vi "InAs-GaAs superlattice-111229a.vi"() -> ()   [LabVIEW 2011]
uses:
  development/wait_globals.vi
panel:
  out "Wait Time Remaining(m:s)":string
  out "Waiting":bool
  out "Total Wait Time (m:s)":string
  out "step number  5":i32
  in  "Number of \nGrowth Steps 5":i32=10
  out "step number  4":i32
  in  "Number of \nGrowth Steps 4":i32=10
  out "step number  3":i32
  in  "Number of \nGrowth Steps 3":i32=10
  out "step number  2":i32
  in  "Number of \nGrowth Steps 2":i32=10
  in  "Ga Flow 1":dbl=5.49
  in  "Indium Flow":dbl=45.0
  in  "Number of \nGrowth Steps":i32=10
  out "step number":i32
  in  "As_Gas Flow":dbl=3.4
  in  "Manifold H2 Flow":dbl=730.0
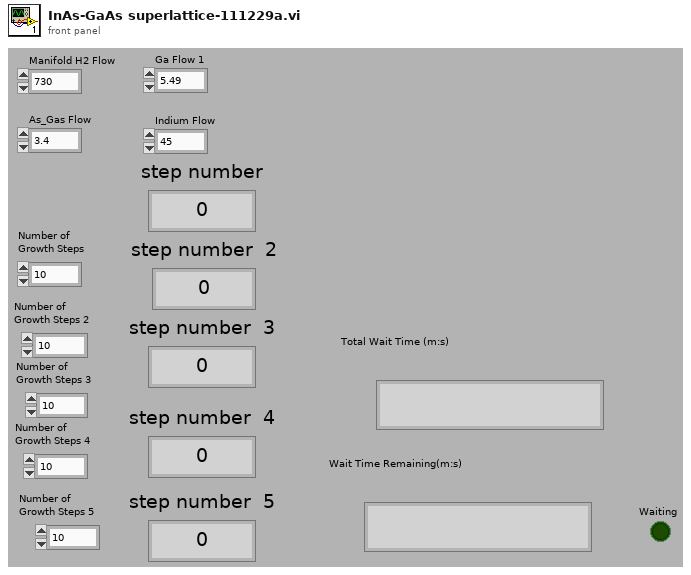
[diagram p1: front panel]
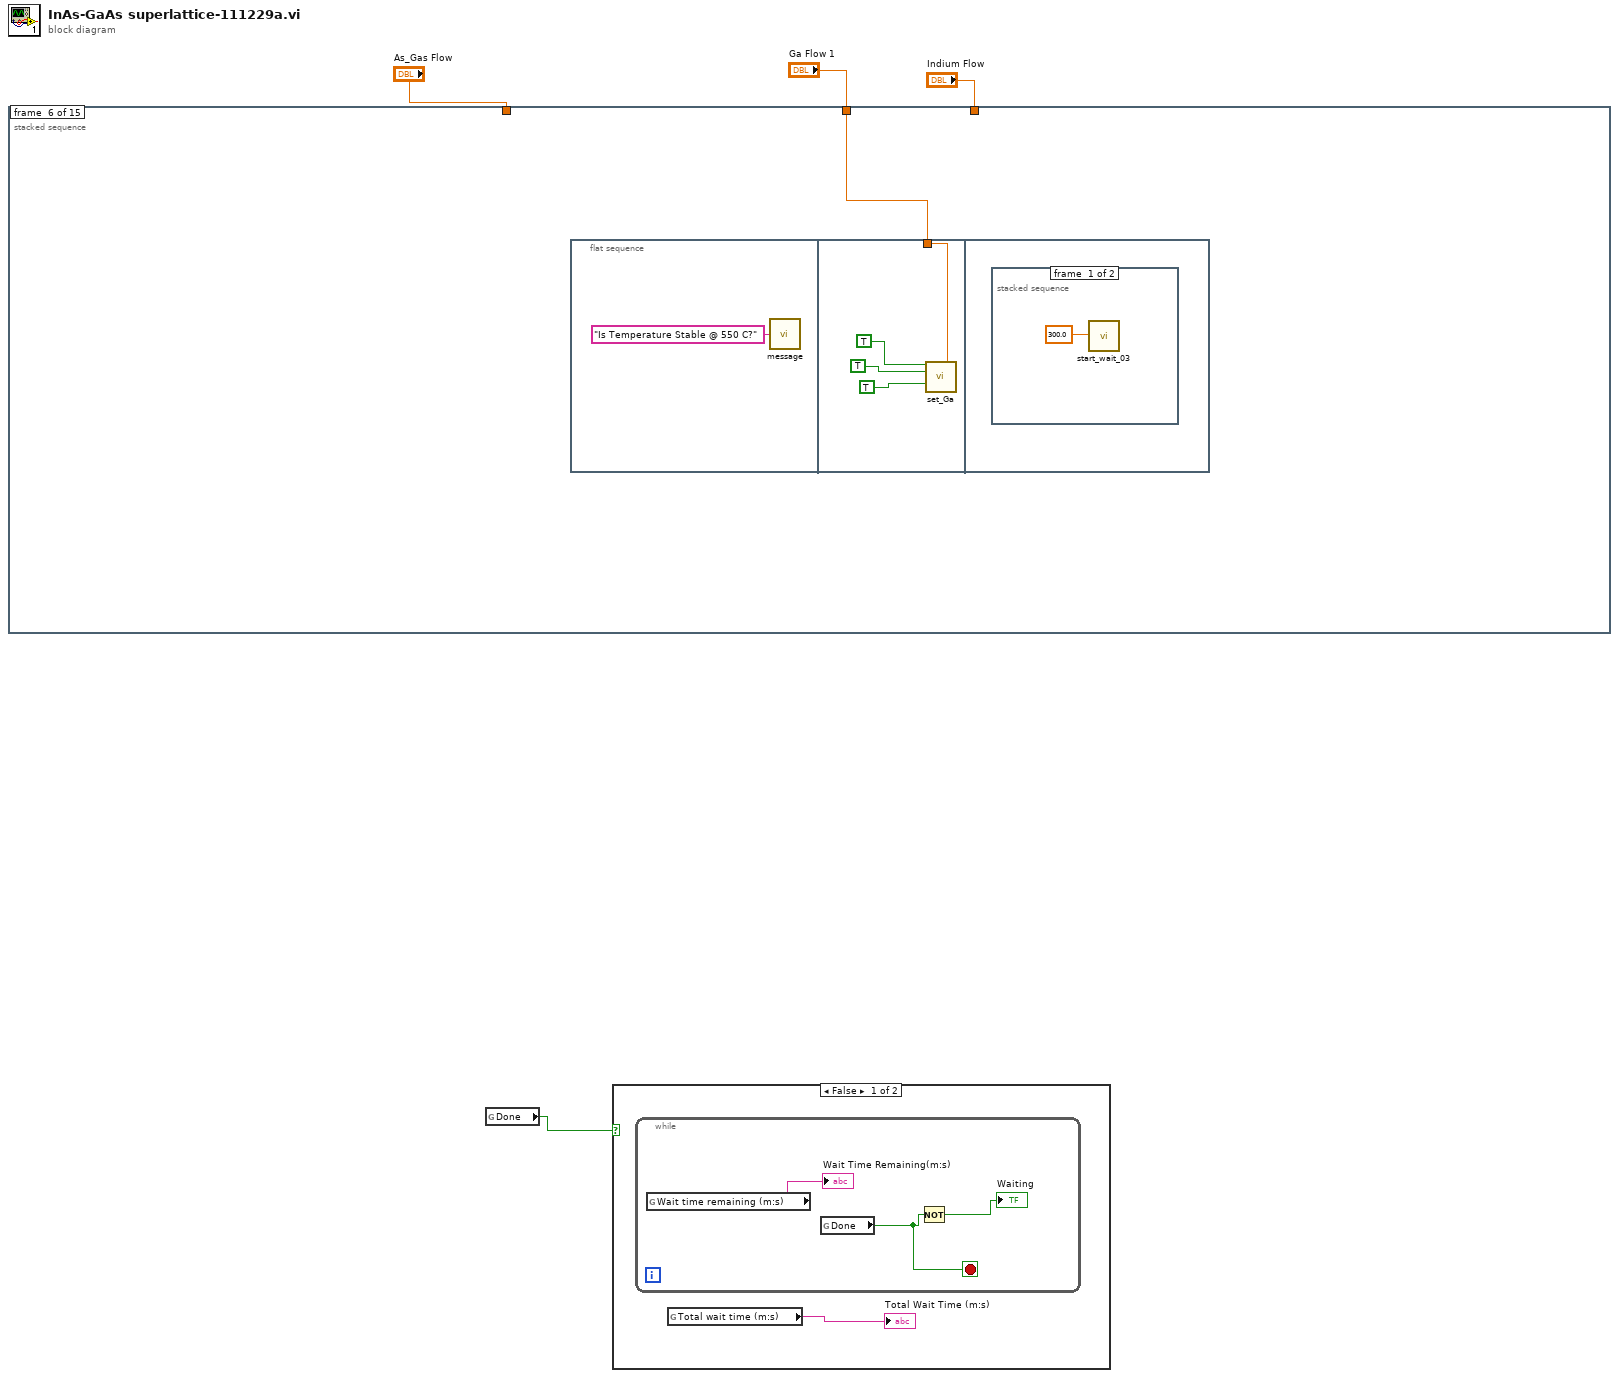
[diagram p0: block diagram]
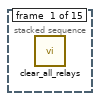
[diagram p3: hidden frame]
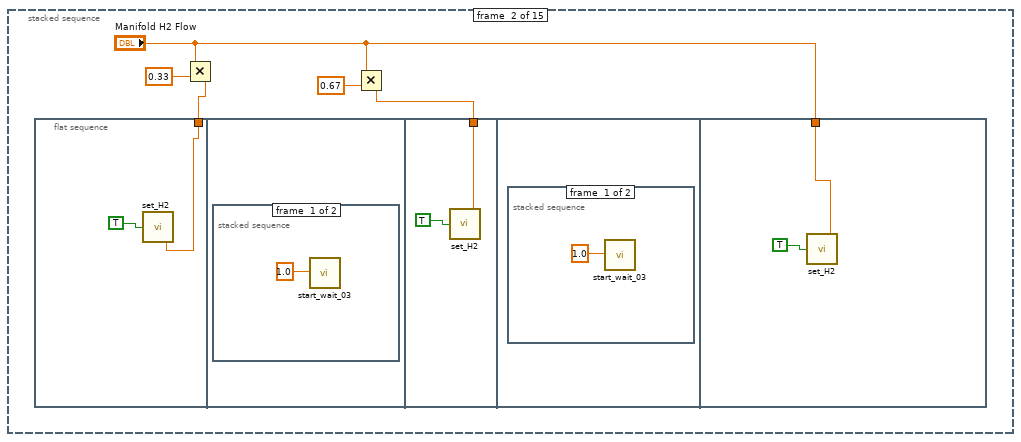
[diagram p4: hidden frame]
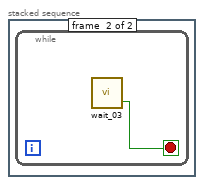
[diagram p5: hidden frame]
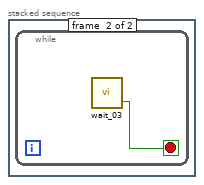
[diagram p6: hidden frame]
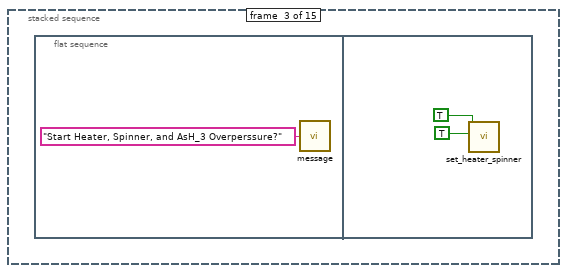
[diagram p7: hidden frame]
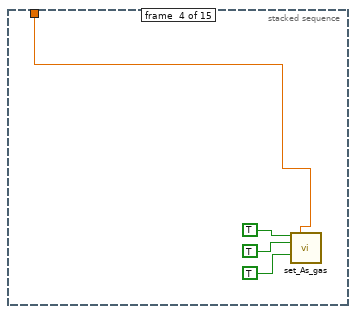
[diagram p8: hidden frame]
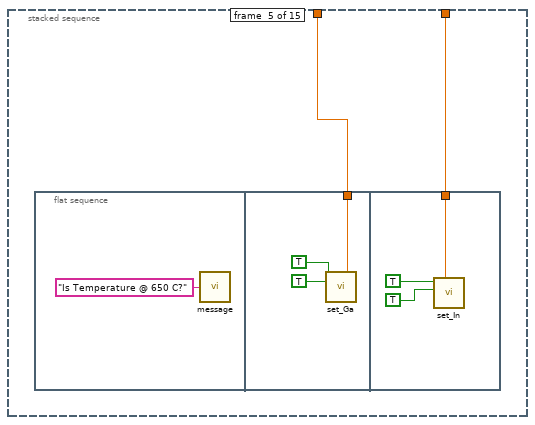
[diagram p9: hidden frame]
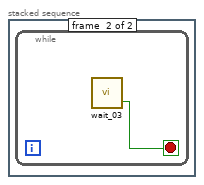
[diagram p10: hidden frame]
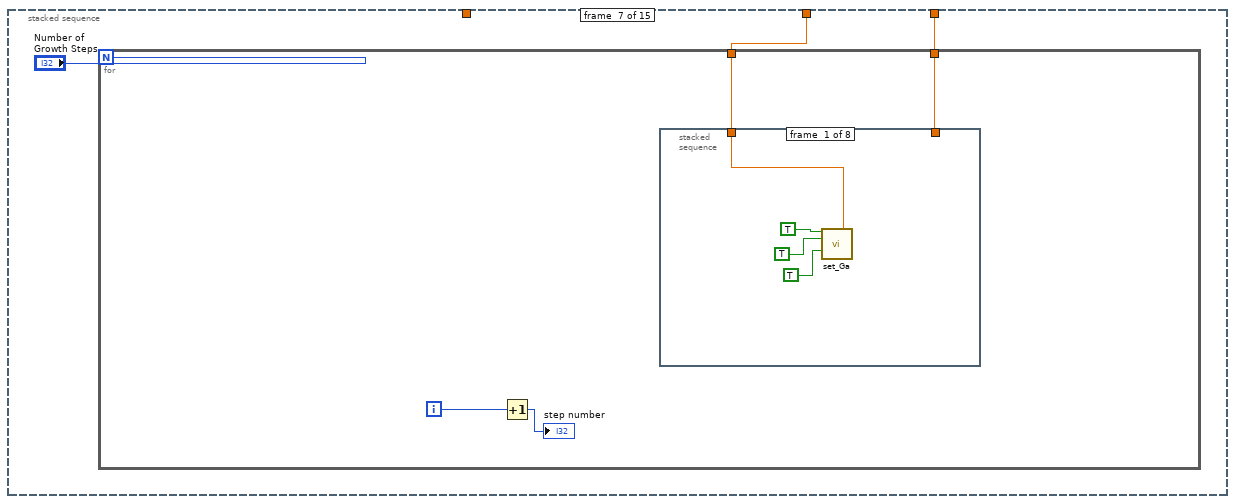
[diagram p11: hidden frame]
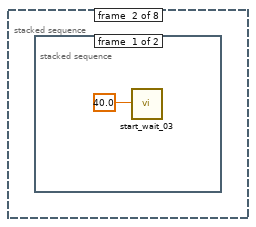
[diagram p12: hidden frame]
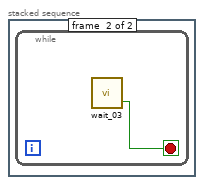
[diagram p13: hidden frame]
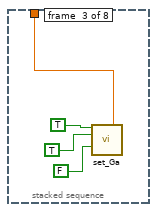
[diagram p14: hidden frame]
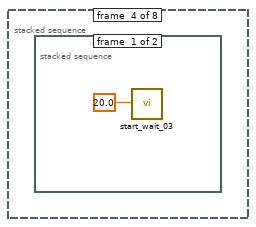
[diagram p15: hidden frame]
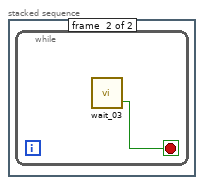
[diagram p16: hidden frame]
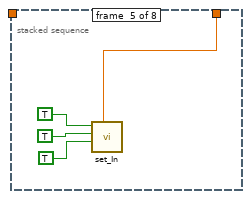
[diagram p17: hidden frame]
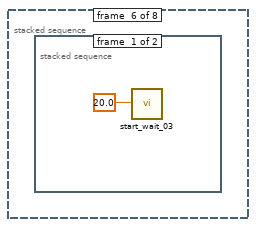
[diagram p18: hidden frame]
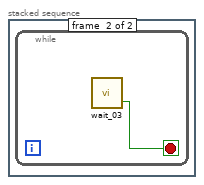
[diagram p19: hidden frame]
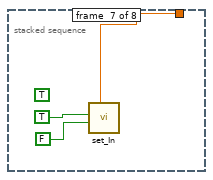
[diagram p20: hidden frame]
diagram:
  n1 = stacked-sequence {
    tunnel: "Ga Flow 1" -> [_ _ _ _ w28 w36 w45 w75 w105 w135 w165 _ _ _ _]
    tunnel: "As_Gas Flow" -> [_ _ _ w23 _ _ _ _ _ _ _ _ _ _ _]
    tunnel: "Indium Flow" -> [_ _ _ _ w27 _ w44 w74 w104 w134 w164 _ _ _ _]
    frame #0 {
      n2 = call "clear_all_relays.vi"() -> ()  [unwired: 2 out]
    }
    frame #1 {
      n3 = flat-sequence {
        tunnel: w9 -> [w10]
        tunnel: w7 -> [w14]
        tunnel: "Manifold H2 Flow" -> [w18]
        frame #0 {
          n4 = call "set_H2.vi"("Manifold H2 Flow"=w10, "H2 Active"=TRUE) -> ()  [unwired: 2 in, 2 out]
        }
        frame #1 {
          n5 = stacked-sequence {
            frame #0 {
              n6 = call "start_wait_03.vi"("Total wait time (s)"=1.0 ("Wait (s)")) -> ()
            }
            frame #1 {
              n7 = while {
                stop <- w13 stop-if-true
                n8 = call "wait_03.vi"() -> ("Done"=w13:bool)  [unwired: 1 in, 1 out]
              }
            }
          }
        }
        frame #2 {
          n9 = call "set_H2.vi"("Manifold H2 Flow"=w14, "H2 Active"=TRUE) -> ()  [unwired: 2 in, 2 out]
        }
        frame #3 {
          n10 = stacked-sequence {
            frame #0 {
              n11 = call "start_wait_03.vi"("Total wait time (s)"=1.0 ("Wait (s)")) -> ()
            }
            frame #1 {
              n12 = while {
                stop <- w17 stop-if-true
                n13 = call "wait_03.vi"() -> ("Done"=w17:bool)  [unwired: 1 in, 1 out]
              }
            }
          }
        }
        frame #4 {
          n14 = call "set_H2.vi"("Manifold H2 Flow"=w18, "H2 Active"=TRUE) -> ()  [unwired: 2 in, 2 out]
        }
      }
      n15 = Multiply(x="Manifold H2 Flow", y=0.33) -> (x*y=w9:dbl)
      n16 = Multiply(x="Manifold H2 Flow", y=0.67) -> (x*y=w7:dbl)
    }
    frame #2 {
      n17 = flat-sequence {
        frame #0 {
          n18 = call "message.vi"("message"="Start Heater, Spinner, and AsH_3 Overperssure?") -> ()
        }
        frame #1 {
          n19 = call "set_heater_spinner.vi"("Spinner"=TRUE, "Heater"=TRUE) -> ()  [unwired: 1 in, 7 out]
        }
      }
    }
    frame #3 {
      n20 = call "set_As_gas.vi"("As_Gas Active"=TRUE, "As_Gas Flow"=w23, "As_Gas In"=TRUE, "As_Gas Run"=TRUE) -> ()  [unwired: 2 in, 10 out]
    }
    frame #4 {
      n21 = flat-sequence {
        tunnel: w28 -> [w30]
        tunnel: w27 -> [w33]
        frame #0 {
          n22 = call "message.vi"("message"="Is Temperature @ 650 C?") -> ()
        }
        frame #1 {
          n23 = call "set_Ga.vi"("Ga Active"=TRUE, "Ga Flow 1"=w30, "Ga Bubbler"=TRUE) -> ()  [unwired: 5 in, 8 out]
        }
        frame #2 {
          n24 = call "set_In.vi"("Indium Flow"=w33, "In Bubbler"=TRUE ("Ga Bubbler"), "In Active"=TRUE ("Ga Active")) -> ()  [unwired: 2 in, 5 out]
        }
      }
    }
    frame #5 {
      n25 = flat-sequence {
        tunnel: w36 -> [w38]
        frame #0 {
          n26 = call "message.vi"("message"="Is Temperature Stable @ 550 C?") -> ()
        }
        frame #1 {
          n27 = call "set_Ga.vi"("Ga Active"=TRUE ("P_Gas Active"), "Ga Flow 1"=w38, "Ga Bubbler"=TRUE ("P_Gas In"), "Ga Run"=TRUE ("P_Gas Run")) -> ()  [unwired: 4 in, 8 out]
        }
        frame #2 {
          n28 = stacked-sequence {
            frame #0 {
              n29 = call "start_wait_03.vi"("Total wait time (s)"=300.0 ("Wait (s)")) -> ()
            }
            frame #1 {
              n30 = while {
                stop <- w43 stop-if-true
                n31 = call "wait_03.vi"() -> ("Done"=w43:bool)  [unwired: 1 in, 1 out]
              }
            }
          }
        }
      }
    }
    frame #6 {
      n32 = for {
        N: "Number of \nGrowth Steps" -> [_]
        tunnel: w45 -> [w48]
        tunnel: w44 -> [w47]
        i -> [w49]
        n33 = Increment(x=w49) -> (x+1=→"step number":i32)
        n34 = stacked-sequence {
          tunnel: w47 -> [_ _ _ _ w63 _ w69 _]
          tunnel: w48 -> [w51 _ w57 _ _ _ _ _]
          frame #0 {
            n35 = call "set_Ga.vi"("Ga Active"=TRUE ("P_Gas Active"), "Ga Flow 1"=w51, "Ga Bubbler"=TRUE ("P_Gas In"), "Ga Run"=TRUE ("P_Gas Run")) -> ()  [unwired: 4 in, 8 out]
          }
          frame #1 {
            n36 = stacked-sequence {
              frame #0 {
                n37 = call "start_wait_03.vi"("Total wait time (s)"=40.0 ("Wait (s)")) -> ()
              }
              frame #1 {
                n38 = while {
                  stop <- w56 stop-if-true
                  n39 = call "wait_03.vi"() -> ("Done"=w56:bool)  [unwired: 1 in, 1 out]
                }
              }
            }
          }
          frame #2 {
            n40 = call "set_Ga.vi"("Ga Active"=TRUE ("P_Gas Active"), "Ga Flow 1"=w57, "Ga Bubbler"=TRUE ("P_Gas In"), "Ga Run"=FALSE ("P_Gas Run")) -> ()  [unwired: 4 in, 8 out]
          }
          frame #3 {
            n41 = stacked-sequence {
              frame #0 {
                n42 = call "start_wait_03.vi"("Total wait time (s)"=20.0 ("Wait (s)")) -> ()
              }
              frame #1 {
                n43 = while {
                  stop <- w62 stop-if-true
                  n44 = call "wait_03.vi"() -> ("Done"=w62:bool)  [unwired: 1 in, 1 out]
                }
              }
            }
          }
          frame #4 {
            n45 = call "set_In.vi"("Indium Flow"=w63, "In Run"=TRUE ("P_Gas Run"), "In Bubbler"=TRUE ("P_Gas In"), "In Active"=TRUE ("P_Gas Active")) -> ()  [unwired: 1 in, 5 out]
          }
          frame #5 {
            n46 = stacked-sequence {
              frame #0 {
                n47 = call "start_wait_03.vi"("Total wait time (s)"=20.0 ("Wait (s)")) -> ()
              }
              frame #1 {
                n48 = while {
                  stop <- w68 stop-if-true
                  n49 = call "wait_03.vi"() -> ("Done"=w68:bool)  [unwired: 1 in, 1 out]
                }
              }
            }
          }
          frame #6 {
            (unwired) TRUE ("P_Gas Active")
            n50 = call "set_In.vi"("Indium Flow"=w69, "In Run"=FALSE ("P_Gas Run"), "In Bubbler"=TRUE ("P_Gas In")) -> ()  [unwired: 2 in, 5 out]
          }
          frame #7 {
            n51 = stacked-sequence {
              frame #0 {
                n52 = call "start_wait_03.vi"("Total wait time (s)"=60.0 ("Wait (s)")) -> ()
              }
              frame #1 {
                n53 = while {
                  stop <- w73 stop-if-true
                  n54 = call "wait_03.vi"() -> ("Done"=w73:bool)  [unwired: 1 in, 1 out]
                }
              }
            }
          }
        }
      }
    }
    frame #7 {
      n55 = for {
        N: "Number of \nGrowth Steps 2" -> [_]
        tunnel: w75 -> [w78]
        tunnel: w74 -> [w77]
        i -> [w79]
        n56 = Increment(x=w79) -> (x+1=→"step number  2":i32)
        n57 = stacked-sequence {
          tunnel: w77 -> [_ _ _ _ w93 _ w99 _]
          tunnel: w78 -> [w81 _ w87 _ _ _ _ _]
          frame #0 {
            n58 = call "set_Ga.vi"("Ga Active"=TRUE ("P_Gas Active"), "Ga Flow 1"=w81, "Ga Bubbler"=TRUE ("P_Gas In"), "Ga Run"=TRUE ("P_Gas Run")) -> ()  [unwired: 4 in, 8 out]
          }
          frame #1 {
            n59 = stacked-sequence {
              frame #0 {
                n60 = call "start_wait_03.vi"("Total wait time (s)"=40.0 ("Wait (s)")) -> ()
              }
              frame #1 {
                n61 = while {
                  stop <- w86 stop-if-true
                  n62 = call "wait_03.vi"() -> ("Done"=w86:bool)  [unwired: 1 in, 1 out]
                }
              }
            }
          }
          frame #2 {
            n63 = call "set_Ga.vi"("Ga Active"=TRUE ("P_Gas Active"), "Ga Flow 1"=w87, "Ga Bubbler"=TRUE ("P_Gas In"), "Ga Run"=FALSE ("P_Gas Run")) -> ()  [unwired: 4 in, 8 out]
          }
          frame #3 {
            n64 = stacked-sequence {
              frame #0 {
                n65 = call "start_wait_03.vi"("Total wait time (s)"=20.0 ("Wait (s)")) -> ()
              }
              frame #1 {
                n66 = while {
                  stop <- w92 stop-if-true
                  n67 = call "wait_03.vi"() -> ("Done"=w92:bool)  [unwired: 1 in, 1 out]
                }
              }
            }
          }
          frame #4 {
            n68 = call "set_In.vi"("Indium Flow"=w93, "In Run"=TRUE ("P_Gas Run"), "In Bubbler"=TRUE ("P_Gas In"), "In Active"=TRUE ("P_Gas Active")) -> ()  [unwired: 1 in, 5 out]
          }
          frame #5 {
            n69 = stacked-sequence {
              frame #0 {
                n70 = call "start_wait_03.vi"("Total wait time (s)"=20.0 ("Wait (s)")) -> ()
              }
              frame #1 {
                n71 = while {
                  stop <- w98 stop-if-true
                  n72 = call "wait_03.vi"() -> ("Done"=w98:bool)  [unwired: 1 in, 1 out]
                }
              }
            }
          }
          frame #6 {
            (unwired) TRUE ("P_Gas Active")
            n73 = call "set_In.vi"("Indium Flow"=w99, "In Run"=FALSE ("P_Gas Run"), "In Bubbler"=TRUE ("P_Gas In")) -> ()  [unwired: 2 in, 5 out]
          }
          frame #7 {
            n74 = stacked-sequence {
              frame #0 {
                n75 = call "start_wait_03.vi"("Total wait time (s)"=60.0 ("Wait (s)")) -> ()
              }
              frame #1 {
                n76 = while {
                  stop <- w103 stop-if-true
                  n77 = call "wait_03.vi"() -> ("Done"=w103:bool)  [unwired: 1 in, 1 out]
                }
              }
            }
          }
        }
      }
    }
    frame #8 {
      n78 = for {
        N: "Number of \nGrowth Steps 3" -> [_]
        tunnel: w105 -> [w108]
        tunnel: w104 -> [w107]
        i -> [w109]
        n79 = Increment(x=w109) -> (x+1=→"step number  3":i32)
        n80 = stacked-sequence {
          tunnel: w107 -> [_ _ _ _ w123 _ w129 _]
          tunnel: w108 -> [w111 _ w117 _ _ _ _ _]
          frame #0 {
            n81 = call "set_Ga.vi"("Ga Active"=TRUE ("P_Gas Active"), "Ga Flow 1"=w111, "Ga Bubbler"=TRUE ("P_Gas In"), "Ga Run"=TRUE ("P_Gas Run")) -> ()  [unwired: 4 in, 8 out]
          }
          frame #1 {
            n82 = stacked-sequence {
              frame #0 {
                n83 = call "start_wait_03.vi"("Total wait time (s)"=40.0 ("Wait (s)")) -> ()
              }
              frame #1 {
                n84 = while {
                  stop <- w116 stop-if-true
                  n85 = call "wait_03.vi"() -> ("Done"=w116:bool)  [unwired: 1 in, 1 out]
                }
              }
            }
          }
          frame #2 {
            n86 = call "set_Ga.vi"("Ga Active"=TRUE ("P_Gas Active"), "Ga Flow 1"=w117, "Ga Bubbler"=TRUE ("P_Gas In"), "Ga Run"=FALSE ("P_Gas Run")) -> ()  [unwired: 4 in, 8 out]
          }
          frame #3 {
            n87 = stacked-sequence {
              frame #0 {
                n88 = call "start_wait_03.vi"("Total wait time (s)"=20.0 ("Wait (s)")) -> ()
              }
              frame #1 {
                n89 = while {
                  stop <- w122 stop-if-true
                  n90 = call "wait_03.vi"() -> ("Done"=w122:bool)  [unwired: 1 in, 1 out]
                }
              }
            }
          }
          frame #4 {
            n91 = call "set_In.vi"("Indium Flow"=w123, "In Run"=TRUE ("P_Gas Run"), "In Bubbler"=TRUE ("P_Gas In"), "In Active"=TRUE ("P_Gas Active")) -> ()  [unwired: 1 in, 5 out]
          }
          frame #5 {
            n92 = stacked-sequence {
              frame #0 {
                n93 = call "start_wait_03.vi"("Total wait time (s)"=20.0 ("Wait (s)")) -> ()
              }
              frame #1 {
                n94 = while {
                  stop <- w128 stop-if-true
                  n95 = call "wait_03.vi"() -> ("Done"=w128:bool)  [unwired: 1 in, 1 out]
                }
              }
            }
          }
          frame #6 {
            (unwired) TRUE ("P_Gas Active")
            n96 = call "set_In.vi"("Indium Flow"=w129, "In Run"=FALSE ("P_Gas Run"), "In Bubbler"=TRUE ("P_Gas In")) -> ()  [unwired: 2 in, 5 out]
          }
          frame #7 {
            n97 = stacked-sequence {
              frame #0 {
                n98 = call "start_wait_03.vi"("Total wait time (s)"=60.0 ("Wait (s)")) -> ()
              }
              frame #1 {
                n99 = while {
                  stop <- w133 stop-if-true
                  n100 = call "wait_03.vi"() -> ("Done"=w133:bool)  [unwired: 1 in, 1 out]
                }
              }
            }
          }
        }
      }
    }
    frame #9 {
      n101 = for {
        N: "Number of \nGrowth Steps 4" -> [_]
        tunnel: w135 -> [w138]
        tunnel: w134 -> [w137]
        i -> [w139]
        n102 = Increment(x=w139) -> (x+1=→"step number  4":i32)
        n103 = stacked-sequence {
          tunnel: w137 -> [_ _ _ _ w153 _ w159 _]
          tunnel: w138 -> [w141 _ w147 _ _ _ _ _]
          frame #0 {
            n104 = call "set_Ga.vi"("Ga Active"=TRUE ("P_Gas Active"), "Ga Flow 1"=w141, "Ga Bubbler"=TRUE ("P_Gas In"), "Ga Run"=TRUE ("P_Gas Run")) -> ()  [unwired: 4 in, 8 out]
          }
          frame #1 {
            n105 = stacked-sequence {
              frame #0 {
                n106 = call "start_wait_03.vi"("Total wait time (s)"=40.0 ("Wait (s)")) -> ()
              }
              frame #1 {
                n107 = while {
                  stop <- w146 stop-if-true
                  n108 = call "wait_03.vi"() -> ("Done"=w146:bool)  [unwired: 1 in, 1 out]
                }
              }
            }
          }
          frame #2 {
            n109 = call "set_Ga.vi"("Ga Active"=TRUE ("P_Gas Active"), "Ga Flow 1"=w147, "Ga Bubbler"=TRUE ("P_Gas In"), "Ga Run"=FALSE ("P_Gas Run")) -> ()  [unwired: 4 in, 8 out]
          }
          frame #3 {
            n110 = stacked-sequence {
              frame #0 {
                n111 = call "start_wait_03.vi"("Total wait time (s)"=20.0 ("Wait (s)")) -> ()
              }
              frame #1 {
                n112 = while {
                  stop <- w152 stop-if-true
                  n113 = call "wait_03.vi"() -> ("Done"=w152:bool)  [unwired: 1 in, 1 out]
                }
              }
            }
          }
          frame #4 {
            n114 = call "set_In.vi"("Indium Flow"=w153, "In Run"=TRUE ("P_Gas Run"), "In Bubbler"=TRUE ("P_Gas In"), "In Active"=TRUE ("P_Gas Active")) -> ()  [unwired: 1 in, 5 out]
          }
          frame #5 {
            n115 = stacked-sequence {
              frame #0 {
                n116 = call "start_wait_03.vi"("Total wait time (s)"=20.0 ("Wait (s)")) -> ()
              }
              frame #1 {
                n117 = while {
                  stop <- w158 stop-if-true
                  n118 = call "wait_03.vi"() -> ("Done"=w158:bool)  [unwired: 1 in, 1 out]
                }
              }
            }
          }
          frame #6 {
            (unwired) TRUE ("P_Gas Active")
            n119 = call "set_In.vi"("Indium Flow"=w159, "In Run"=FALSE ("P_Gas Run"), "In Bubbler"=TRUE ("P_Gas In")) -> ()  [unwired: 2 in, 5 out]
          }
          frame #7 {
            n120 = stacked-sequence {
              frame #0 {
                n121 = call "start_wait_03.vi"("Total wait time (s)"=60.0 ("Wait (s)")) -> ()
              }
              frame #1 {
                n122 = while {
                  stop <- w163 stop-if-true
                  n123 = call "wait_03.vi"() -> ("Done"=w163:bool)  [unwired: 1 in, 1 out]
                }
              }
            }
          }
        }
      }
    }
    frame #10 {
      n124 = for {
        N: "Number of \nGrowth Steps 5" -> [_]
        tunnel: w165 -> [w167]
        tunnel: w164 -> [w168]
        i -> [w169]
        n125 = Increment(x=w169) -> (x+1=→"step number  5":i32)
        n126 = stacked-sequence {
          tunnel: w168 -> [_ _ _ _ w183 _ w189 _]
          tunnel: [_ _ _ _ _ _ w189 _] -> _
          tunnel: w167 -> [w171 _ w177 _ _ _ _ _]
          frame #0 {
            n127 = call "set_Ga.vi"("Ga Active"=TRUE ("P_Gas Active"), "Ga Flow 1"=w171, "Ga Bubbler"=TRUE ("P_Gas In"), "Ga Run"=TRUE ("P_Gas Run")) -> ()  [unwired: 4 in, 8 out]
          }
          frame #1 {
            n128 = stacked-sequence {
              frame #0 {
                n129 = call "start_wait_03.vi"("Total wait time (s)"=40.0 ("Wait (s)")) -> ()
              }
              frame #1 {
                n130 = while {
                  stop <- w176 stop-if-true
                  n131 = call "wait_03.vi"() -> ("Done"=w176:bool)  [unwired: 1 in, 1 out]
                }
              }
            }
          }
          frame #2 {
            n132 = call "set_Ga.vi"("Ga Active"=TRUE ("P_Gas Active"), "Ga Flow 1"=w177, "Ga Bubbler"=TRUE ("P_Gas In"), "Ga Run"=FALSE ("P_Gas Run")) -> ()  [unwired: 4 in, 8 out]
          }
          frame #3 {
            n133 = stacked-sequence {
              frame #0 {
                n134 = call "start_wait_03.vi"("Total wait time (s)"=20.0 ("Wait (s)")) -> ()
              }
              frame #1 {
                n135 = while {
                  stop <- w182 stop-if-true
                  n136 = call "wait_03.vi"() -> ("Done"=w182:bool)  [unwired: 1 in, 1 out]
                }
              }
            }
          }
          frame #4 {
            n137 = call "set_In.vi"("Indium Flow"=w183, "In Run"=TRUE ("P_Gas Run"), "In Bubbler"=TRUE ("P_Gas In"), "In Active"=TRUE ("P_Gas Active")) -> ()  [unwired: 1 in, 5 out]
          }
          frame #5 {
            n138 = stacked-sequence {
              frame #0 {
                n139 = call "start_wait_03.vi"("Total wait time (s)"=20.0 ("Wait (s)")) -> ()
              }
              frame #1 {
                n140 = while {
                  stop <- w188 stop-if-true
                  n141 = call "wait_03.vi"() -> ("Done"=w188:bool)  [unwired: 1 in, 1 out]
                }
              }
            }
          }
          frame #6 {
            (unwired) TRUE ("P_Gas Active")
            n142 = call "set_In.vi"("Indium Flow"=w189, "In Run"=FALSE ("P_Gas Run"), "In Bubbler"=TRUE ("P_Gas In")) -> ()  [unwired: 2 in, 5 out]
          }
          frame #7 {
            n143 = stacked-sequence {
              frame #0 {
                n144 = call "start_wait_03.vi"("Total wait time (s)"=60.0 ("Wait (s)")) -> ()
              }
              frame #1 {
                n145 = while {
                  stop <- w193 stop-if-true
                  n146 = call "wait_03.vi"() -> ("Done"=w193:bool)  [unwired: 1 in, 1 out]
                }
              }
            }
          }
        }
      }
    }
    frame #11 {
      n147 = flat-sequence {
        frame #0 {
          n148 = call "set_heater_spinner.vi"("Spinner"=TRUE ("Ga Active")) -> ()  [unwired: 2 in, 7 out]
        }
        frame #1 {
          n149 = call "set_Ga.vi"("Ga Active"=TRUE, "Ga Flow 1"=10.0) -> ()  [unwired: 6 in, 8 out]
        }
        frame #2 {
          n150 = call "set_In.vi"("Indium Flow"=100.0 ("Aluminum Flow"), "In Active"=TRUE ("Ga Active")) -> ()  [unwired: 3 in, 5 out]
        }
        frame #3 {
          n151 = stacked-sequence {
            frame #0 {
              n152 = call "start_wait_03.vi"("Total wait time (s)"=20.0 ("Wait (s)")) -> ()
            }
            frame #1 {
              n153 = while {
                stop <- w200 stop-if-true
                n154 = call "wait_03.vi"() -> ("Done"=w200:bool)  [unwired: 1 in, 1 out]
              }
            }
          }
        }
      }
    }
    frame #12 {
      n155 = flat-sequence {
        frame #0 {
          n156 = call "set_Ga.vi"("Ga Remote"=FALSE) -> ()  [unwired: 7 in, 8 out]
        }
        frame #1 {
          n157 = call "set_In.vi"("In Run"=FALSE ("Ga Remote")) -> ()  [unwired: 4 in, 5 out]
        }
        frame #2 {
          n158 = call "message.vi"("message"="Is Temperature < 300C?") -> ()
        }
      }
    }
    frame #13 {
      n159 = call "set_As_gas.vi"("As_Gas Remote"=FALSE) -> ()  [unwired: 5 in, 10 out]
    }
    frame #14 {
      n160 = flat-sequence {
        frame #0 {
          n161 = call "message.vi"("message"="Is Temperarure < 100C?") -> ()
        }
        frame #1 {
          n162 = call "set_heater_spinner.vi"("Heater/Spinner Remote"=FALSE) -> ()  [unwired: 2 in, 7 out]
        }
        frame #2 {
          n163 = call "set_H2.vi"("H2N2 Remote"=FALSE) -> ()  [unwired: 3 in, 2 out]
        }
      }
    }
  }
  n164 = global read "wait_globals.vi" "Done"() -> (w1:bool)
  n165 = case shown="False" w1 {
    frame False {
      n166 = global read "wait_globals.vi" "Total wait time (m:s)"() -> (→"Total Wait Time (m:s)":string)
    }
    frame True {
    }
  }
  n167 = while {
    stop <- w209 stop-if-true
    n168 = global read "wait_globals.vi" "Wait time remaining (m:s)"() -> (→"Wait Time Remaining(m:s)":string)
    n169 = global read "wait_globals.vi" "Done"() -> (w209:bool)
    n170 = Not(x=w209) -> (.not. x?=→"Waiting":bool)
  }
